vi "Teleop.vi"(10 "Match Info":T3={"Autonomous Elapsed Seconds"=0.0, "TeleOp Elapsed Seconds"=0.0, "Disabled Elapsed Seconds"=0.0, "Visited Autonomous"=FALSE, "Visited TeleOp"=FALSE, "Visited Disabled"=FALSE, "Autonomous Settings"={"Autonomous Style"=enum."Independent", "VI Refnum"=refnum}}, 11 "Call Context":T4) -> ()   [LabVIEW 2019]
doc: "This VI is called for each TeleOp packet received from the DS where the robot is not disabled. It is often used to read from the joysticks and update I/O or to update setpoints for timed control loops. It should complete and return within 20 milliseconds or it may miss DS packets."
uses:
  <vilib>/Rock Robotics/WPI/DriverStation/WPI_DriverStationDerivedRobotMode.ctl
  <vilib>/Rock Robotics/WPI/DriverStation/WPI_DriverStationMatch Info.ctl
  <vilib>/Rock Robotics/WPI/ThirdParty/Phoenix-LabVIEW/Motor Controller/Controls/CTRE_Phoenix_MotorControl_ControlMode.ctl
  <vilib>/Rock Robotics/WPI/Utilities/WPI_GetSetVariantRefNum.vi
  Toolbox/Piston/Piston Toggle.vi
  <vilib>/Rock Robotics/WPI/Solenoid/WPI_SolenoidSetEnum.vi
  <vilib>/Rock Robotics/WPI/ThirdParty/Phoenix-LabVIEW/Motor Controller/Get/CTRE_Phoenix_MotorController_GetSupplyAndStatorCurrent_Enhanced.vi
  <vilib>/Rock Robotics/WPI/ThirdParty/Phoenix-LabVIEW/Motor Controller/Get/CTRE_Phoenix_MotorController_GetSelectedSensorData.vi
  <vilib>/addons/control/pid/NI_PID_pid.lvlib
  <vilib>/Rock Robotics/Network Tables/NT Write Number.vi
  <vilib>/addons/control/pid/pid.llb/PID (DBL).vi
  <vilib>/Rock Robotics/Network Tables/NT Read Number.vi
panel:
  out "Gear Ratio":dbl
  in  "I Zone":dbl=1000.0
  in  "Bypass":bool
  in  "output rate (Joystick Percentage/Second)":dbl=140.0 format="%.2f"
  in  "Vertical (Y) Multiplier":dbl=0.7
  in  "Horizontal (X) Multiplier":dbl=0.45
  out "Raw Units":i32
  out "Output RPM":dbl=1.0
  in  "F":dbl=0.0461
  in  "D":dbl
  in  "I":dbl=0.001
  in  "P":dbl=0.1
  in  "Set PIDF":bool=TRUE
  out "Output":bool
  out "Shooter Motor Current 2":T1(graph)
  in  "Setpoint RPM":dbl=7000.0
  out "Rpm":dbl(graph)
  in  "Power Min":dbl
  in  "Magazine Power":dbl=0.25
  in  "Magazine Overflow Power":dbl=-1.0
  in  "Magazine Intake Power":dbl=0.25
  in  "Intake power":dbl=0.7
  out "tx":dbl
  in  "PID gains":T2={"proportional gain (Kc)"=0.025, "integral time (Ti, min)"=0.01, "derivative time (Td, min)"=0.0} {"derivative time (Td, min)" format="%.3g"; "integral time (Ti, min)" format="%.3e"; "proportional gain (Kc)" format="%.3g"}
  in  "Winch Power":dbl=1.0
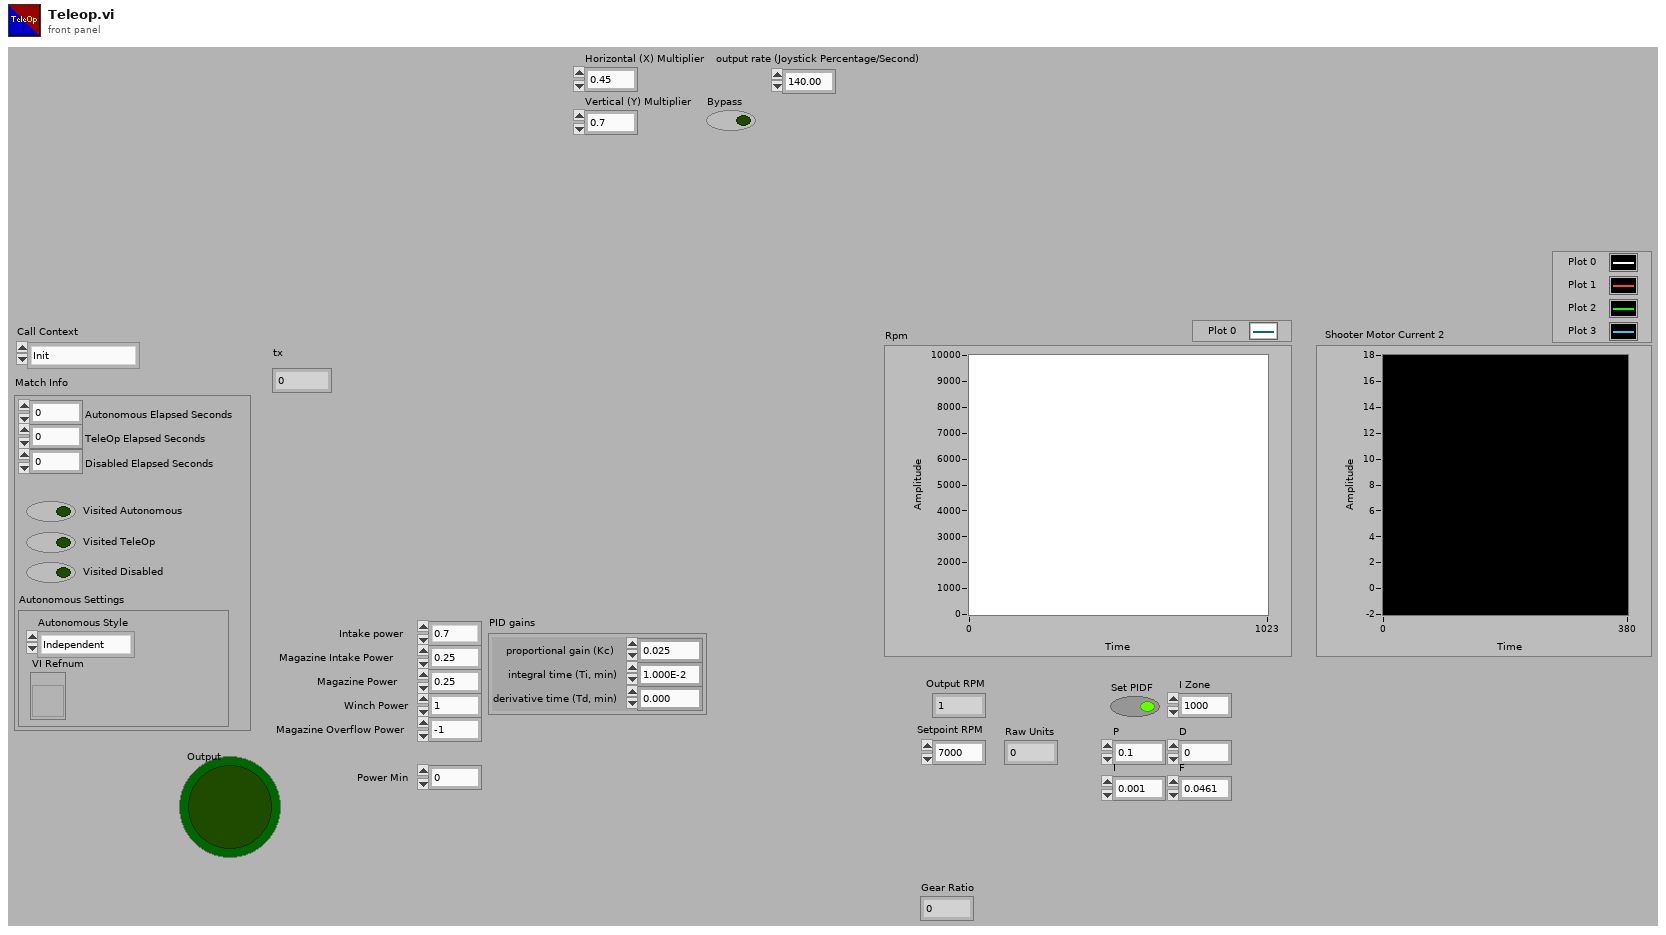
[diagram p1: front panel]
types:
  T1 = cluster{"Supply Current":dbl, "Stator Current":dbl, "Supply Current":dbl, "Stator Current":dbl}
  T2 = cluster{"proportional gain (Kc)":dbl, "integral time (Ti, min)":dbl, "derivative time (Td, min)":dbl}
  T3 = typedef "WPI_DriverStationMatch Info.ctl" = cluster{"Autonomous Elapsed Seconds":dbl, "TeleOp Elapsed Seconds":dbl, "Disabled Elapsed Seconds":dbl, "Visited Autonomous":bool, "Visited TeleOp":bool, "Visited Disabled":bool, "Autonomous Settings":cluster{"Autonomous Style":enum16{"Iterative", "Independent"}, "VI Refnum":refnum<vi>}}
  T4 = typedef "WPI_DriverStationDerivedRobotMode.ctl" = enum16{"Init", "Execute", "Stop"}
  T5 = typedef "CTRE_Phoenix_MotorControl_ControlMode.ctl" = u16
  T6 = cluster{"Intake In":bool, "Intake Out":bool, "Magazine In":bool, "Magazine Out":bool, "Winch In":bool, "Winch Out":bool, "Climber Hold":bool, "Intake Pistons":bool, "Shooter Hold":bool, "None":bool, "Power Toggle":bool, "Auto Target":bool}
  T7 = typedef "WPI_JoystickDevRef.ctl" = cluster{"Device":T8}
  T8 = typedef "WPI_JoystickDeviceEnum.ctl" = enum16{"USB 0", "USB 1", "USB 2", "USB 3", "USB 4", "USB 5"}
  T9 = typedef "WPI_MotorControlDeviceRef.ctl" = cluster{"DeviceStatus":errorcluster, "Type":T10, "PWM":cluster{"PWM Channel":T11, "DeadBand":T12}, "CAN":cluster{"Device Number":u8, "SetOutput VI Ref":variant, "GetOutput VI Ref":variant, "Enable VI Ref":variant, "Disable VI Ref":variant, "Data":variant}, "Invert":bool, "DIO PWM":cluster{"PWM \"Enable\" Channel":T11, "DIOChannel":T13, "PWM Rate":dbl}}
  T10 = typedef "WPI_MotorControlType.ctl" = enum16{"PWM", "CAN", "DIO PWM"}
  T11 = typedef "FPGA_DIOPWMChannel.ctl" = enum8{"PWM 0", "PWM 1", "PWM 2", "PWM 3", "PWM 4", "PWM 5", "PWM 6", "PWM 7", "PWM 8", "PWM 9", "PWM MXP 0", "PWM MXP 1", "PWM MXP 2", "PWM MXP 3", "PWM MXP 4", "PWM MXP 5", "PWM MXP 6", "PWM MXP 7", "PWM MXP 8", "PWM MXP 9", "Invalid"}
  T12 = typedef "WPI_PWMDeadband.ctl" = cluster{"Name":string, "maxPositivePwm":i32, "minPositivePwm":i32, "centerPwm":i32, "maxNegativePwm":i32, "minNegativePwm":i32, "angularRange":u16}
  T13 = typedef "FPGA_DIOChannel.ctl" = enum8{"DIO 0", "DIO 1", "DIO 2", "DIO 3", "DIO 4", "DIO 5", "DIO 6", "DIO 7", "DIO 8", "DIO 9", "DIO MXP 0", "DIO MXP 1", "DIO MXP 2", "DIO MXP 3", "DIO MXP 4", "DIO MXP 5", "DIO MXP 6", "DIO MXP 7", "DIO MXP 8", "DIO MXP 9", "DIO MXP 10", "DIO MXP 11", "DIO MXP 12", "DIO MXP 13", "DIO MXP 14", "DIO MXP 15", "SPI Port CS1", "SPI Port CS2", "SPI Port CS3", "SPI Port MISO", "SPI Port MOSI", "Invalid"}
  T14 = typedef "WPI_SolenoidValue.ctl" = enum16{"Off", "On", "Forward", "Reverse"}
  T15 = typedef "WPI_SolenoidDevRef.ctl" = cluster{"DevStatus":errorcluster, "Pneumatics Control Module":u8, "Forward Solenoid Channel":T16, "Reverse Solenoid Channel":T16}
  T16 = typedef "WPI_SolenoidChannel.ctl" = enum8{"Solenoid 0", "Solenoid 1", "Solenoid 2", "Solenoid 3", "Solenoid 4", "Solenoid 5", "Solenoid 6", "Solenoid 7", "Invalid"}
  T17 = typedef "WPI_DigitalInputDevRef.ctl" = cluster{"DevStatus":errorcluster, "DIO Channel":T13}
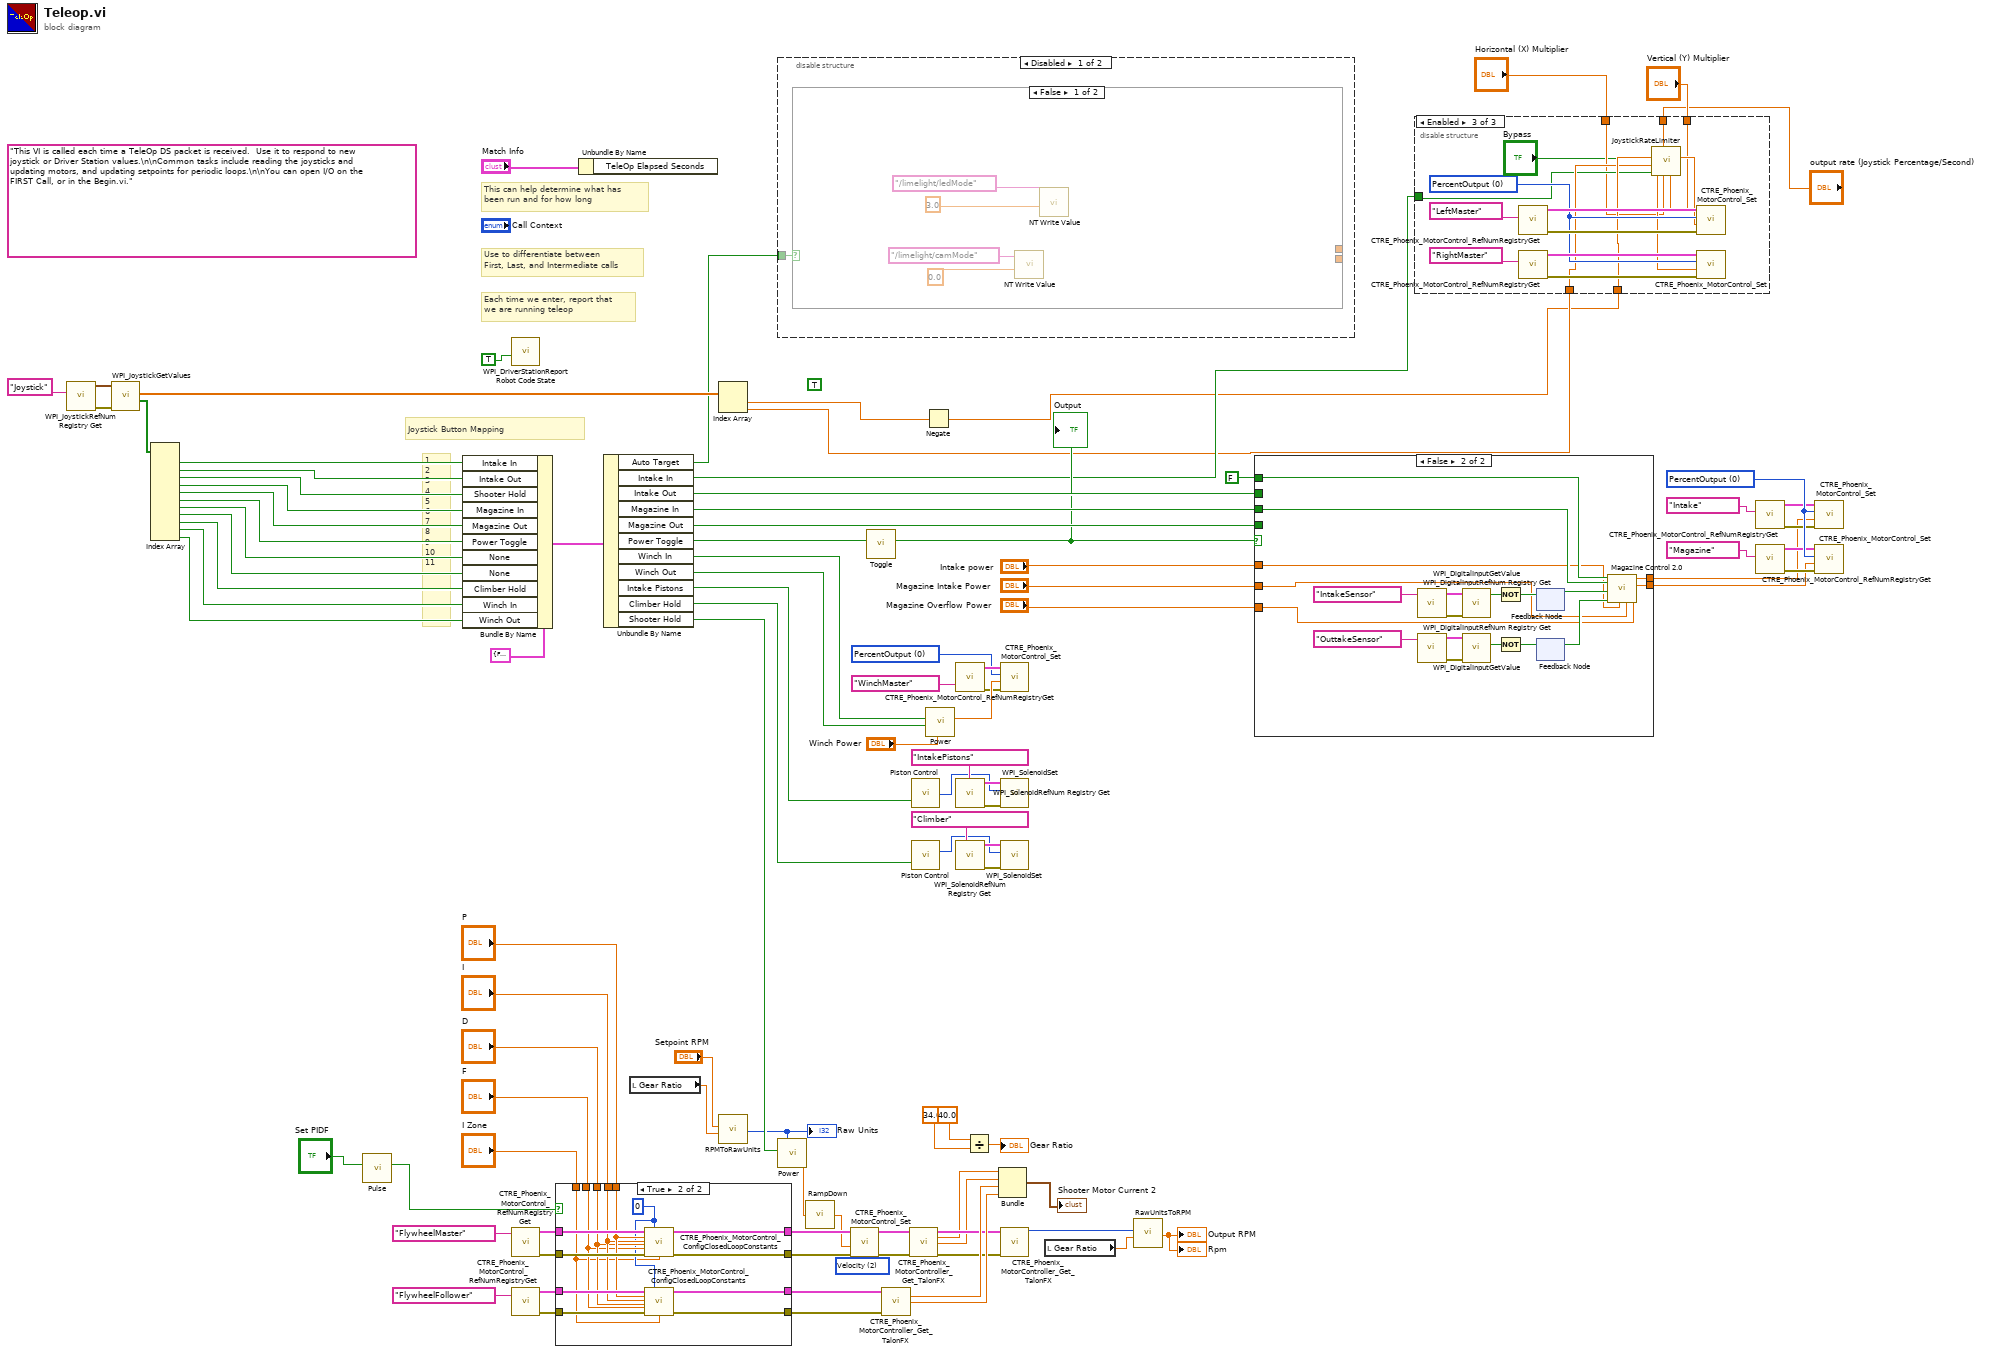
[diagram p0: block diagram]
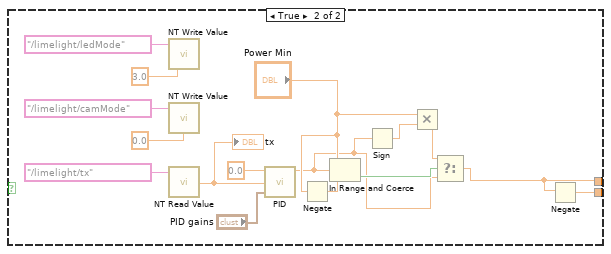
[diagram p2: hidden frame]
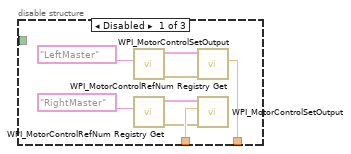
[diagram p5: hidden frame]
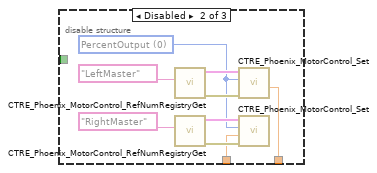
[diagram p6: hidden frame]
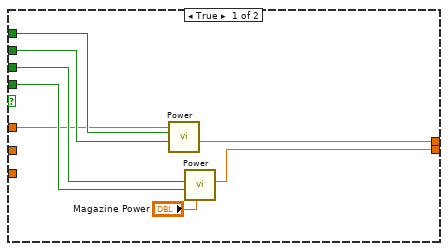
[diagram p7: hidden frame]
diagram:
  w44 = T5 2 items=["PercentOutput"=0, "Position"=1, "Velocity"=2, "Current"=3, "Follower"=5, "MotionProfile"=6, "MotionMagic"=7, "MotionProfileArc"=10, "Disabled"=15] ("Control Mode")
  w57 = T5 0 items=["PercentOutput"=0, "Position"=1, "Velocity"=2, "Current"=3, "Follower"=5, "MotionProfile"=6, "MotionMagic"=7, "MotionProfileArc"=10, "Disabled"=15] ("Control Mode")
  w60 = T5 0 items=["PercentOutput"=0, "Position"=1, "Velocity"=2, "Current"=3, "Follower"=5, "MotionProfile"=6, "MotionMagic"=7, "MotionProfileArc"=10, "Disabled"=15] ("Control Mode")
  (unwired) TRUE ("Square Inputs")
  (unwired) "This VI is called each time a TeleOp DS packet is received.  Use it to respond to new joystick or Driver Station values.\n\nCommon tasks include reading the joysticks and updating motors, and updating setpoints for periodic loops.\n\nYou can open I/O on the FIRST Call, or in the Begin.vi."
  # "1\n2\n3\n4\n5\n6\n7\n8\n9\n10\n11"
  # "Joystick Button Mapping"
  # "Each time we enter, report that\nwe are running teleop"
  # "Use to differentiate between\nFirst, Last, and Intermediate calls"
  # "This can help determine what has\nbeen run and for how long"
  n1 = call <vilib>:"WPI_JoystickRefNum Registry Get.vi"("refnum name"="Joystick") -> ("error out"=w101:errorcluster, "JoystickDevRef"=w100:T7)  [unwired: 9 in]
  n2 = call <vilib>:"WPI_JoystickGetValues.vi"("error in (no error)"=w101, "JoystickDevRef"=w100) -> ("Buttons"=w87:bool[], "Axes"=w98:dbl[])  [unwired: 5 in, 3 out]
  n3 = Index Array(array=w87) -> (element #1=w88:bool, element #2=w64:bool, element #3=w96:bool, element #4=w65:bool, element #5=w95:bool, element #6=w94:bool, element #7=w93:bool, element #8=w92:bool, element #9=w91:bool, element #10=w90:bool, element #11=w89:bool)  [unwired: 11 in]
  n4 = call "Pulse.vi"("Input"="Set PIDF") -> ("Output"=w29:bool)  [unwired: 10 in]
  n5 = Bundle By Name(cluster=T6 {"Intake In"=FALSE, "Intake Out"=FALSE, "Magazine In"=FALSE, "Magazine Out"=FALSE, "Winch In"=FALSE, "Winch Out"=FALSE, "Climber Hold"=FALSE, "Intake Pistons"=FALSE, "Shooter Hold"=FALSE, "None"=FALSE, "Power Toggle"=FALSE, "Auto Target"=FALSE} ("input cluster"), "Intake In"=w88, "Intake Out"=w64, "Shooter Hold"=w96, "Magazine In"=w65, "Magazine Out"=w95, "Power Toggle"=w94, "None"=w93, "None"=w92, "Climber Hold"=w91, "Winch In"=w90, "Winch Out"=w89) -> (w86:T6)
  n6 = call <vilib>:"WPI_DriverStationReport Robot Code State.vi"("TeleOp"=TRUE ("Autonomous")) -> ()  [unwired: 10 in, 1 out]
  n7 = call <vilib>:"CTRE_Phoenix_MotorControl_RefNumRegistryGet.vi"("refnum name"="FlywheelMaster") -> ("error out"=w33:errorcluster, "PhoenixMotorControlDevRef"=w34:T9)  [unwired: 9 in]
  n8 = call <vilib>:"CTRE_Phoenix_MotorControl_RefNumRegistryGet.vi"("refnum name"="FlywheelFollower") -> ("error out"=w31:errorcluster, "PhoenixMotorControlDevRef"=w32:T9)  [unwired: 9 in]
  n9 = case shown="True" w29 {
    tunnel: w34 -> [w107 w121]
    tunnel: w33 -> [w106 w120]
    tunnel: w32 -> [w105 w119]
    tunnel: w31 -> [w104 w118]
    tunnel: "P" -> [_ w117]
    tunnel: "I" -> [_ w116]
    tunnel: "D" -> [_ w115]
    tunnel: "F" -> [_ w114]
    tunnel: [w107 w112] -> w8
    tunnel: [w106 w111] -> w7
    tunnel: [w105 w109] -> w24
    tunnel: [w104 w110] -> w23
    tunnel: "I Zone" -> [_ w108]
    frame False {
    }
    frame True {
      w113 = 0 ("slotIdx")
      n10 = call <vilib>:"CTRE_Phoenix_MotorControl_ConfigClosedLoopConstants.vi"("PhoenixMotorControlDevRef"=w121, "slotIdx"=w113, "P"=w117, "I"=w116, "D"=w115, "error in (no error)"=w120, "F"=w114, "I Zone"=w108) -> ("PhoenixMotorControlDevRef"=w112:T9, "error out"=w111:errorcluster)  [unwired: 6 in]
      n11 = call <vilib>:"CTRE_Phoenix_MotorControl_ConfigClosedLoopConstants.vi"("PhoenixMotorControlDevRef"=w119, "slotIdx"=w113, "P"=w117, "I"=w116, "D"=w115, "error in (no error)"=w118, "F"=w114, "I Zone"=w108) -> ("PhoenixMotorControlDevRef"=w109:T9, "error out"=w110:errorcluster)  [unwired: 6 in]
    }
  }
  n12 = Unbundle By Name("Match Info") -> ()  [unwired: 1 out]
  n13 = Unbundle By Name(w86) -> ("Auto Target"=w74:bool, "Intake In"=w17:bool, "Intake Out"=w85:bool, "Magazine In"=w84:bool, "Magazine Out"=w83:bool, "Power Toggle"=w59:bool, "Winch In"=w82:bool, "Winch Out"=w81:bool, "Intake Pistons"=w71:bool, "Climber Hold"=w70:bool, "Shooter Hold"=w48:bool)
  n14 = local read "Gear Ratio"() -> (w3:dbl)
  n15 = Index Array(array=w98) -> (element #1=w15:dbl, element #2=w14:dbl)  [unwired: 2 in]
  n16 = call "RPMToRawUnits.vi"("Gear Ratio"=w3, "RPM"="Setpoint RPM") -> ("Raw Units"=w1:i32)  [unwired: 9 in]
  "Raw Units" <- w1
  n17 = disable-structure shown="Disabled" {
    disable-tunnel: w74 -> [w122 _]
    frame Disabled {
      n18 = case shown="False" w122 {
        tunnel: [_ w128] -> _
        tunnel: [_ w139] -> _
        frame False {
          n19 = call-poly <vilib>:"NT Write Value.vi"("Numeric"=0.0, "Name"="/limelight/camMode") -> ()  [unwired: 9 in, 1 out]
          n20 = call-poly <vilib>:"NT Write Value.vi"("Numeric"=3.0, "Name"="/limelight/ledMode") -> ()  [unwired: 9 in, 1 out]
        }
        frame True {
          n21 = call-poly <vilib>:"NT Write Value.vi"("Numeric"=3.0, "Name"="/limelight/ledMode") -> ()  [unwired: 9 in, 1 out]
          n22 = call-poly <vilib>:"NT Write Value.vi"("Numeric"=0.0, "Name"="/limelight/camMode") -> ()  [unwired: 9 in, 1 out]
          n23 = call-poly <vilib>:"NT Read Value.vi"("Name"="/limelight/tx") -> ("Numeric"=w132:dbl)  [unwired: 9 in, 1 out]
          "tx" <- w132
          n24 = call-poly <vilib>:"PID.vi"("PID gains"="PID gains", "process variable"=w132, "setpoint"=0.0) -> ("output"=w127:dbl)  [unwired: 7 in, 1 out]
          n25 = Negate(x="Power Min") -> (-x=w134:dbl)
          n26 = In Range and Coerce(upper limit="Power Min", x=w127, lower limit=w134) -> (In Range?=w133:bool)  [unwired: 1 out]
          n27 = Sign(1:w127) -> (0:w131:dbl)
          n28 = Multiply(x="Power Min", y=w131) -> (x*y=w129:dbl)
          n29 = Select(t=w129, s=w133, f=w127) -> (s? t:f=w128:dbl)
          n30 = Negate(x=w128) -> (-x=w139:dbl)
        }
      }
    }
    frame Enabled {
    }
  }
  n31 = call "Power.vi"("Positive Power"=w1, "Positive"=w48) -> ("Output"=w6:dbl)  [unwired: 9 in]
  n32 = call "RampDown.vi"("Output"=w6) -> ("Numeric"=w5:dbl)
  n33 = call <vilib>:"CTRE_Phoenix_MotorControl_Set.vi"("error in (no error)"=w7, "Output"=w5, "Control Mode"=w44, "PhoenixMotorControlDevRef"=w8) -> ("error out"=w20:errorcluster, "PhoenixMotorControlDevRef"=w21:T9)  [unwired: 6 in]
  n34 = call "Toggle.vi"("Input"=w59) -> ("Output"=w47:bool)  [unwired: 10 in]
  "Output" <- w47
  n35 = call-poly <vilib>:"CTRE_Phoenix_MotorController_Get_TalonFX.vi"("PhoenixMotorControlDevRef"=w24, "error in"=w23) -> ("Supply Current"=w43:dbl, "Stator Current"=w42:dbl)  [unwired: 10 in, 2 out]
  n36 = call-poly <vilib>:"CTRE_Phoenix_MotorController_Get_TalonFX.vi"("PhoenixMotorControlDevRef"=w21, "error in"=w20) -> ("PhoenixMotorControlDevRef"=w39:T9, "Supply Current"=w37:dbl, "Stator Current"=w36:dbl, "error out"=w38:errorcluster)  [unwired: 10 in]
  n37 = call-poly "Piston Control.vi"("Input"=w71) -> ("Output"=w73:T14)  [unwired: 1 in]
  n38 = call-poly "Piston Control.vi"("Input"=w70) -> ("Output"=w72:T14)  [unwired: 1 in]
  n39 = Negate(x=w15) -> (-x=w13:dbl)
  n40 = call "Power.vi"("Positive Power"="Winch Power", "Negative"=w81, "Positive"=w82) -> ("Output"=w97:dbl)  [unwired: 8 in]
  n41 = call <vilib>:"CTRE_Phoenix_MotorControl_RefNumRegistryGet.vi"("refnum name"="WinchMaster") -> ("error out"=w62:errorcluster, "PhoenixMotorControlDevRef"=w61:T9)  [unwired: 9 in]
  n42 = call <vilib>:"WPI_SolenoidRefNum Registry Get.vi"("refnum name"="IntakePistons") -> ("error out"=w80:errorcluster, "SolenoidDevRef"=w79:T15)  [unwired: 9 in]
  n43 = call <vilib>:"WPI_SolenoidRefNum Registry Get.vi"("refnum name"="Climber") -> ("error out"=w77:errorcluster, "SolenoidDevRef"=w76:T15)  [unwired: 9 in]
  n44 = Divide(x=40.0, y=34.0) -> (x/y=→"Gear Ratio":dbl)
  n45 = Bundle("Supply Current"=w37, "Stator Current"=w36, "Supply Current"=w43, "Stator Current"=w42) -> (→"Shooter Motor Current 2":T1)  [unwired: 1 in]
  n46 = call <vilib>:"CTRE_Phoenix_MotorControl_Set.vi"("error in (no error)"=w62, "Output"=w97, "Control Mode"=w60, "PhoenixMotorControlDevRef"=w61) -> ()  [unwired: 6 in, 2 out]
  n47 = call-poly <vilib>:"WPI_SolenoidSet.vi"("error in (no error)"=w80, "Value"=w73, "SolenoidDevRef"=w79) -> ()  [unwired: 7 in, 2 out]
  n48 = call-poly <vilib>:"WPI_SolenoidSet.vi"("error in (no error)"=w77, "Value"=w72, "SolenoidDevRef"=w76) -> ()  [unwired: 7 in, 2 out]
  n49 = call-poly <vilib>:"CTRE_Phoenix_MotorController_Get_TalonFX.vi"("PhoenixMotorControlDevRef"=w39, "error in"=w38) -> ("Velocity (Raw Sensor Units per 100 ms)"=w35:i32)  [unwired: 10 in, 3 out]
  n50 = local read "Gear Ratio"() -> (w2:dbl)
  n51 = call "RawUnitsToRPM.vi"("Gear Ratio"=w2, "Raw Units"=w35) -> ("RPM"=→"Rpm" →"Output RPM":dbl)  [unwired: 9 in]
  n52 = case shown="False" w47 {
    tunnel: w85 -> [w150 _]
    tunnel: w84 -> [w149 w156]
    tunnel: w83 -> [w148 _]
    tunnel: FALSE ("Intake In") -> [w147 w159]
    tunnel: [w145 w152] -> w50
    tunnel: [w146 w151] -> w49
    tunnel: "Magazine Overflow Power" -> [_ w153]
    tunnel: "Magazine Intake Power" -> [_ w154]
    tunnel: "Intake power" -> [w144 w155]
    frame True {
      n53 = call "Power.vi"("Positive Power"=w144, "Negative"=w150, "Positive"=w147) -> ("Output"=w145:dbl)  [unwired: 8 in]
      n54 = call "Power.vi"("Positive Power"="Magazine Power", "Negative"=w148, "Positive"=w149) -> ("Output"=w146:dbl)  [unwired: 8 in]
    }
    frame False {
      n55 = call <vilib>:"WPI_DigitalInputRefNum Registry Get.vi"("refnum name"="IntakeSensor") -> ("error out"=w169:errorcluster, "DigitalInputDevRef"=w168:T17)  [unwired: 9 in]
      n56 = call <vilib>:"WPI_DigitalInputRefNum Registry Get.vi"("refnum name"="OuttakeSensor") -> ("error out"=w166:errorcluster, "DigitalInputDevRef"=w167:T17)  [unwired: 9 in]
      n57 = call <vilib>:"WPI_DigitalInputGetValue.vi"("error in (no error)"=w169, "DigitalInputDevRef"=w168) -> ("Value"=w165:bool)  [unwired: 7 in, 2 out]
      n58 = call <vilib>:"WPI_DigitalInputGetValue.vi"("error in (no error)"=w166, "DigitalInputDevRef"=w167) -> ("Value"=w164:bool)  [unwired: 7 in, 2 out]
      n59 = Not(x=w165) -> (.not. x?=w161:bool)
      n60 = Not(x=w164) -> (.not. x?=w160:bool)
      n61 = feedback-in #1(w161) -> ()
      n62 = feedback #1() -> (w157:bool)  [unwired: 1 in]
      n63 = feedback #2() -> (w158:bool)  [unwired: 1 in]
      n64 = feedback-in #2(w160) -> ()
      n65 = call "Magazine Control 2.0.vi"("Magazine Overflow Power"=w153, "Magazine Power"=w154, "Intake Power"=w155, "Outtake Sensor"=w158, "Intake Sensor"=w157, "Outtake Button"=w156, "Intake Button"=w159) -> ("Magazine"=w151:dbl, "Intake"=w152:dbl)  [unwired: 3 in]
    }
  }
  n66 = disable-structure shown="Enabled" {
    disable-tunnel: w13 -> [w177 w179 w195]
    disable-tunnel: w14 -> [w176 w178 w194]
    disable-tunnel: w17 -> [_ _ w191]
    disable-tunnel: "Horizontal (X) Multiplier" -> [_ _ w190]
    disable-tunnel: "Vertical (Y) Multiplier" -> [_ _ w189]
    disable-tunnel: "output rate (Joystick Percentage/Second)" -> [_ _ w188]
    frame Disabled {
      n67 = call <vilib>:"WPI_MotorControlRefNum Registry Get.vi"("refnum name"="LeftMaster") -> ("error out"=w173:errorcluster, "MotorControlDevRef"=w172:T9)  [unwired: 9 in]
      n68 = call <vilib>:"WPI_MotorControlRefNum Registry Get.vi"("refnum name"="RightMaster") -> ("error out"=w171:errorcluster, "MotorControlDevRef"=w170:T9)  [unwired: 9 in]
      n69 = call <vilib>:"WPI_MotorControlSetOutput.vi"("error in (no error)"=w173, "Output"=w177, "MotorControlDevRef"=w172) -> ()  [unwired: 6 in, 3 out]
      n70 = call <vilib>:"WPI_MotorControlSetOutput.vi"("error in (no error)"=w171, "Output"=w176, "MotorControlDevRef"=w170) -> ()  [unwired: 6 in, 3 out]
    }
    frame Disabled {
      w180 = T5 0 items=["PercentOutput"=0, "Position"=1, "Velocity"=2, "Current"=3, "Follower"=5, "MotionProfile"=6, "MotionMagic"=7, "MotionProfileArc"=10, "Disabled"=15] ("Control Mode")
      n71 = call <vilib>:"CTRE_Phoenix_MotorControl_RefNumRegistryGet.vi"("refnum name"="LeftMaster") -> ("error out"=w184:errorcluster, "PhoenixMotorControlDevRef"=w183:T9)  [unwired: 9 in]
      n72 = call <vilib>:"CTRE_Phoenix_MotorControl_RefNumRegistryGet.vi"("refnum name"="RightMaster") -> ("error out"=w182:errorcluster, "PhoenixMotorControlDevRef"=w181:T9)  [unwired: 9 in]
      n73 = call <vilib>:"CTRE_Phoenix_MotorControl_Set.vi"("error in (no error)"=w184, "Output"=w179, "Control Mode"=w180, "PhoenixMotorControlDevRef"=w183) -> ()  [unwired: 6 in, 2 out]
      n74 = call <vilib>:"CTRE_Phoenix_MotorControl_Set.vi"("error in (no error)"=w182, "Output"=w178, "Control Mode"=w180, "PhoenixMotorControlDevRef"=w181) -> ()  [unwired: 6 in, 2 out]
    }
    frame Enabled {
      w196 = T5 0 items=["PercentOutput"=0, "Position"=1, "Velocity"=2, "Current"=3, "Follower"=5, "MotionProfile"=6, "MotionMagic"=7, "MotionProfileArc"=10, "Disabled"=15] ("Control Mode")
      n75 = call <vilib>:"CTRE_Phoenix_MotorControl_RefNumRegistryGet.vi"("refnum name"="LeftMaster") -> ("error out"=w200:errorcluster, "PhoenixMotorControlDevRef"=w199:T9)  [unwired: 9 in]
      n76 = call <vilib>:"CTRE_Phoenix_MotorControl_RefNumRegistryGet.vi"("refnum name"="RightMaster") -> ("error out"=w198:errorcluster, "PhoenixMotorControlDevRef"=w197:T9)  [unwired: 9 in]
      n77 = call "JoystickRateLimiter.vi"("Vertical (Y) Multiplier"=w189, "Horizontal (X) Multiplier"=w190, "output rate (Joystick Percentage/Second)"=w188, "Direction Toggle"=w191, "Y Input"=w194, "X Input"=w195, "Bypass"="Bypass") -> ("Left Motor Value"=w192:dbl, "Right Motor Value"=w193:dbl)  [unwired: 3 in]
      n78 = call <vilib>:"CTRE_Phoenix_MotorControl_Set.vi"("error in (no error)"=w200, "Output"=w193, "Control Mode"=w196, "PhoenixMotorControlDevRef"=w199) -> ()  [unwired: 6 in, 2 out]
      n79 = call <vilib>:"CTRE_Phoenix_MotorControl_Set.vi"("error in (no error)"=w198, "Output"=w192, "Control Mode"=w196, "PhoenixMotorControlDevRef"=w197) -> ()  [unwired: 6 in, 2 out]
    }
  }
  n80 = call <vilib>:"CTRE_Phoenix_MotorControl_RefNumRegistryGet.vi"("refnum name"="Intake") -> ("error out"=w53:errorcluster, "PhoenixMotorControlDevRef"=w54:T9)  [unwired: 9 in]
  n81 = call <vilib>:"CTRE_Phoenix_MotorControl_RefNumRegistryGet.vi"("refnum name"="Magazine") -> ("error out"=w55:errorcluster, "PhoenixMotorControlDevRef"=w56:T9)  [unwired: 9 in]
  n82 = call <vilib>:"CTRE_Phoenix_MotorControl_Set.vi"("error in (no error)"=w53, "Output"=w50, "Control Mode"=w57, "PhoenixMotorControlDevRef"=w54) -> ()  [unwired: 6 in, 2 out]
  n83 = call <vilib>:"CTRE_Phoenix_MotorControl_Set.vi"("error in (no error)"=w55, "Output"=w49, "Control Mode"=w57, "PhoenixMotorControlDevRef"=w56) -> ()  [unwired: 6 in, 2 out]
